vi "Factory1_Main.vi"() -> ()   [LabVIEW 2020]
uses:
  VdDigitalControl_DAQmx_class/VdDigitalControl_DAQmx.lvclass
  VdDigitalControl_AdvantechADAM_class/VdDigitalControl_AdvantechADAM.lvclass
  VdDigitalControl_Simulated_class/VdDigitalControl_Simulated.lvclass
  VdAnalogInput_Simulated_class/VdAnalogInput_Simulated.lvclass
  VdAnalogInput_DAQmx_class/VdAnalogInput_DAQmx.lvclass
  VdDigitalControl_class/VdDigitalControl.lvclass
  VdAnalogInput_class/VdAnalogInput.lvclass
  VdInstrument_class/VdInstrument.lvclass
panel:
  out "Voltages":cluster{"[0]":dbl, "[1]":dbl}(graph)
  out "error out":errorcluster
  out "CurrentState":bool[](array[boolean])
  # "<< Pump\n<< Fan"
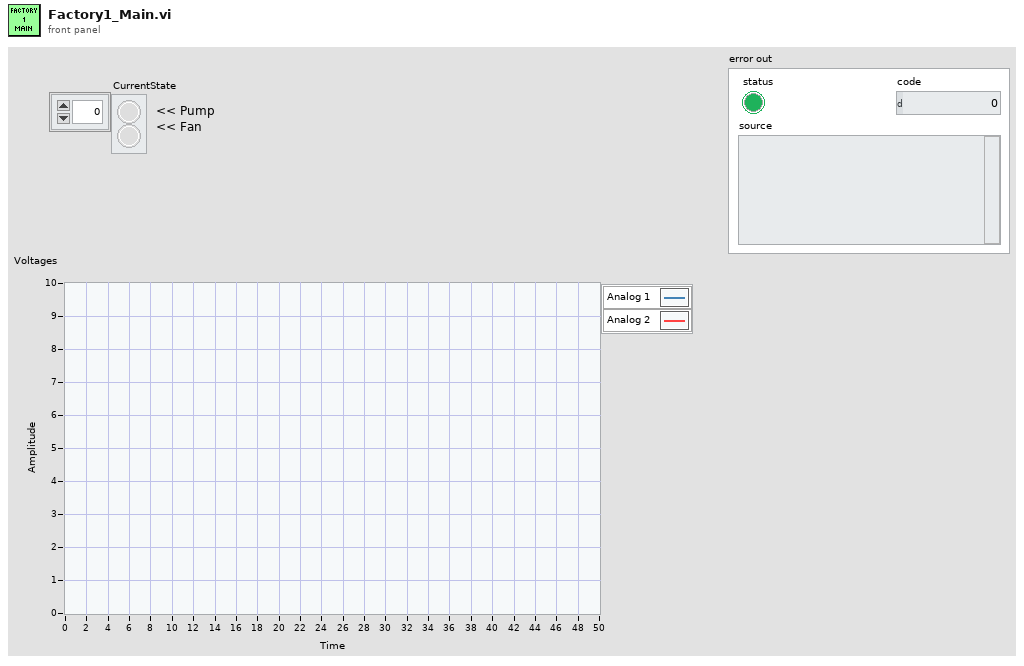
[diagram p1: front panel]
types:
  T1 = cluster{"VdDigitalControl_DAQmx":refnum<class "VdDigitalControl_DAQmx.lvclass">, "VdDigitalControl_AdvantechADAM":refnum<class "VdDigitalControl_AdvantechADAM.lvclass">, "VdDigitalControl_Simulated":refnum<class "VdDigitalControl_Simulated.lvclass">, "VdAnalogInput_Simulated":refnum<class "VdAnalogInput_Simulated.lvclass">, "VdAnalogInput_DAQmx":refnum<class "VdAnalogInput_DAQmx.lvclass">}
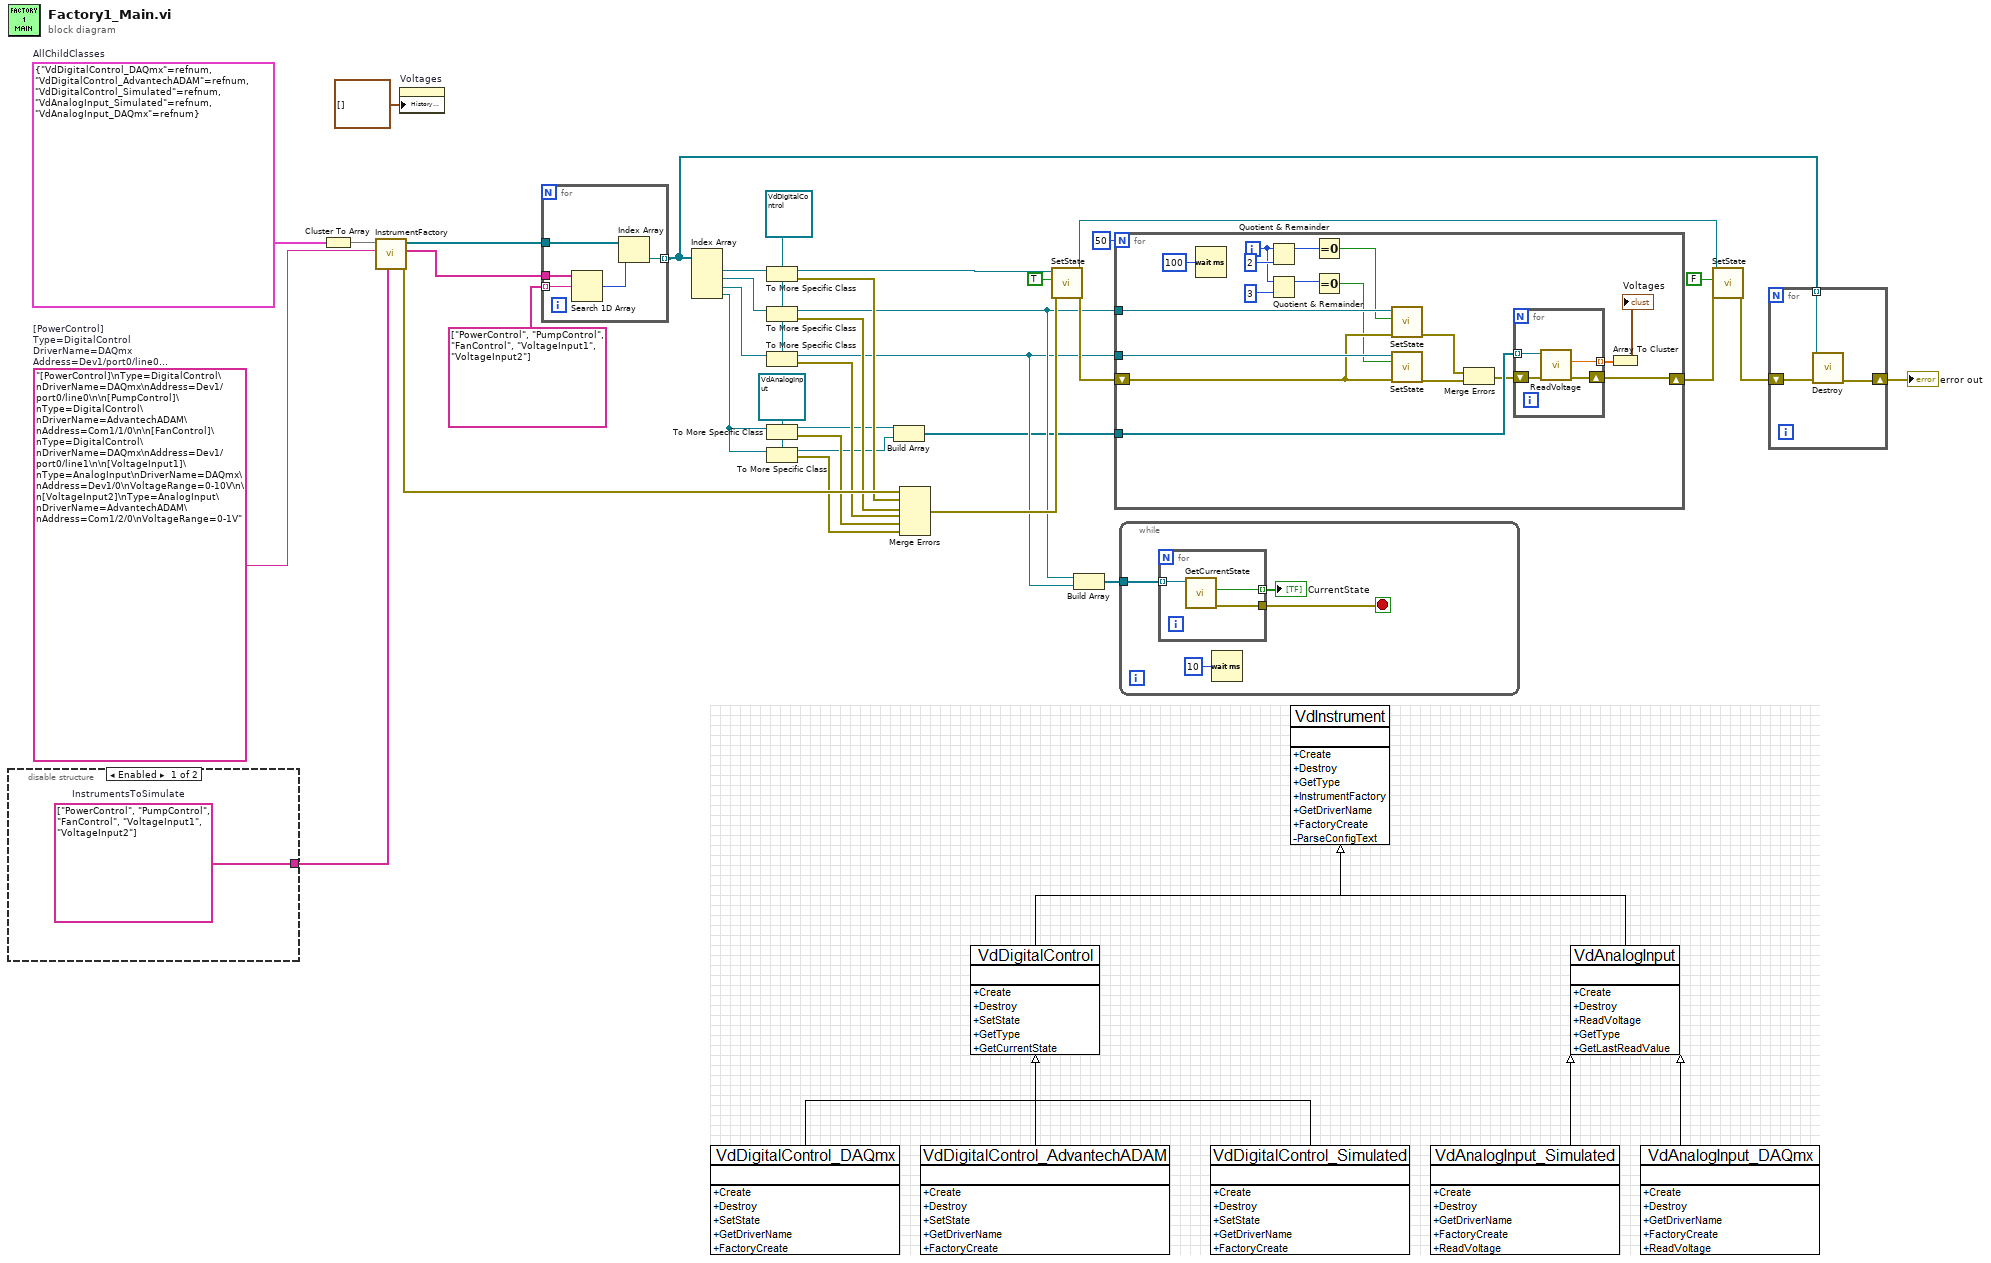
[diagram p0: block diagram]
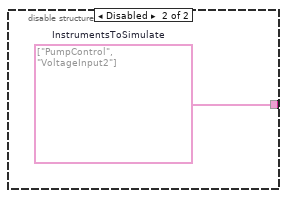
[diagram p2: hidden frame]
diagram:
  w11 = refnum<class "VdAnalogInput.lvclass"> refnum ("VdAnalogInput")
  w25 = refnum<class "VdDigitalControl.lvclass"> refnum ("VdDigitalControl")
  w35 = "[PowerControl]\nType=DigitalControl\nDriverName=DAQmx\nAddress=Dev1/port0/line0\n\n[PumpControl]\nType=DigitalControl\nDriverName=AdvantechADAM\nAddress=Com1/1/0\n\n[FanControl]\nType=DigitalControl\nDriverName=DAQmx\nAddress=Dev1/port0/line1\n\n[VoltageInput1]\nType=AnalogInput\nDriverName=DAQmx\nAddress=Dev1/0\nVoltageRange=0-10V\n\n[VoltageInput2]\nType=AnalogInput\nDriverName=AdvantechADAM\nAddress=Com1/2/0\nVoltageRange=0-1V"  # [PowerControl] Type=DigitalControl DriverName=DAQmx Address=Dev1/port0/line0  [PumpControl] Type=DigitalControl DriverName=AdvantechADAM Address=Com1/1/0  [FanControl] Type=DigitalControl DriverName=DAQmx Address=Dev1/port0/line1  [VoltageInput1] Type=AnalogInput DriverName=DAQmx Address=Dev1/0 VoltageRange=0-10V  [VoltageInput2] Type=AnalogInput DriverName=AdvantechADAM Address=Com1/2/0 VoltageRange=0-1V
  w36 = T1 {"VdDigitalControl_DAQmx"=refnum, "VdDigitalControl_AdvantechADAM"=refnum, "VdDigitalControl_Simulated"=refnum, "VdAnalogInput_Simulated"=refnum, "VdAnalogInput_DAQmx"=refnum}  # AllChildClasses
  n1 = disable-structure shown="Enabled" {
    disable-tunnel: [w38 w39] -> w34
    frame Enabled {
      w38 = string[] ["PowerControl", "PumpControl", "FanControl", "VoltageInput1", "VoltageInput2"]  # InstrumentsToSimulate
    }
    frame Disabled {
      w39 = string[] ["PumpControl", "VoltageInput2"]  # InstrumentsToSimulate
    }
  }
  n2 = Cluster To Array(cluster=w36) -> (array=w37:refnum<class "VdInstrument.lvclass">[])
  n3 = call "InstrumentFactory.vi"("InstrumentsToSimulate"=w34, "InstrumentConfig(ini)"=w35, "AllInstrumentDriver"=w37) -> ("error out"=w23:errorcluster, "InstrumentNamesCreated"=w32:string[], "InstrumentCreated"=w33:refnum<class "VdInstrument.lvclass">[])  [unwired: 6 in]
  n4 = property on="Voltages" class="WFChart (strict)"("History Data"=cluster{"[0]":dbl, "[1]":dbl}[] []) -> ()  [unwired: 2 in, 2 out]
  n5 = for {
    tunnel: w33 -> [w44]
    tunnel: w32 -> [w43]
    tunnel: string[] ["PowerControl", "PumpControl", "FanControl", "VoltageInput1", "VoltageInput2"] -> [w41] mode=indexing
    tunnel: [w40] -> w14 mode=indexing
    n6 = Search 1D Array(1D array=w43, element=w41) -> (index of element=w42:i32)  [unwired: 1 in]
    n7 = Index Array(array=w44, index=w42) -> (element=w40:refnum<class "VdInstrument.lvclass">)
  }
  n8 = Index Array(array=w14) -> (element #1=w30:refnum<class "VdInstrument.lvclass">, element #2=w29:refnum<class "VdInstrument.lvclass">, element #3=w26:refnum<class "VdInstrument.lvclass">, element #4=w12:refnum<class "VdInstrument.lvclass">)  [unwired: 4 in]
  n9 = To More Specific Class(target class=w25, reference=w30) -> (specific class reference=w28:refnum<class "VdDigitalControl.lvclass">, error out=w21:errorcluster)  [unwired: 1 in]
  n10 = To More Specific Class(target class=w25, reference=w29) -> (specific class reference=w17:refnum<class "VdDigitalControl.lvclass">, error out=w20:errorcluster)  [unwired: 1 in]
  n11 = To More Specific Class(target class=w25, reference=w26) -> (specific class reference=w16:refnum<class "VdDigitalControl.lvclass">, error out=w19:errorcluster)  [unwired: 1 in]
  n12 = To More Specific Class(target class=w11, reference=w12) -> (specific class reference=w8:refnum<class "VdAnalogInput.lvclass">, error out=w10:errorcluster)  [unwired: 1 in]
  n13 = To More Specific Class(target class=w11, reference=w12) -> (specific class reference=w7:refnum<class "VdAnalogInput.lvclass">, error out=w9:errorcluster)  [unwired: 1 in]
  n14 = Build Array(w8, w7) -> (w6:refnum<class "VdAnalogInput.lvclass">[])
  n15 = Merge Errors(w23, w21, w20, w19, w10, w9) -> (w22:errorcluster)
  n16 = call-dynamic "SetState.vi"("Error In"=w22, "State"=TRUE, "reference in"=w28) -> ("Error Out"=w24:errorcluster, "reference in"=w1:refnum<class "VdDigitalControl.lvclass">)  [unwired: 7 in]
  n17 = Build Array(w17, w16) -> (w15:refnum<class "VdDigitalControl.lvclass">[])
  n18 = for {
    N: 50 -> [_]
    tunnel: w17 -> [w62]
    tunnel: w16 -> [w61]
    shift-right: [w49] -> w4
    shift-left: w24 -> [w60]
    tunnel: w6 -> [w53]
    i -> [w48]
    n19 = Wait (ms)(milliseconds to wait=u32 100) -> ()  [unwired: 1 out]
    n20 = Quotient & Remainder(x=w48, y=2) -> (x-y*floor(x/y)=w55:i32)  [unwired: 1 out]
    n21 = Quotient & Remainder(x=w48, y=3) -> (x-y*floor(x/y)=w46:i32)  [unwired: 1 out]
    n22 = Equal To 0?(x=w55) -> (x = 0?=w54:bool)
    n23 = Equal To 0?(x=w46) -> (x = 0?=w45:bool)
    n24 = call-dynamic "SetState.vi"("Error In"=w60, "State"=w54, "reference in"=w62) -> ("Error Out"=w57:errorcluster)  [unwired: 7 in, 1 out]
    n25 = call-dynamic "SetState.vi"("Error In"=w60, "State"=w45, "reference in"=w61) -> ("Error Out"=w58:errorcluster)  [unwired: 7 in, 1 out]
    n26 = Merge Errors(w57, w58) -> (w52:errorcluster)
    n27 = for {
      tunnel: w53 -> [w66] mode=indexing
      shift-right: [w64] -> w49
      shift-left: w52 -> [w65]
      tunnel: [w63] -> w51 mode=indexing
      n28 = call-dynamic "ReadVoltage.vi"("Error In"=w65, "reference in"=w66) -> ("Error Out"=w64:errorcluster, "Voltage"=w63:dbl)  [unwired: 7 in, 1 out]
    }
    n29 = Array To Cluster(array=w51) -> (cluster=→"Voltages":cluster{"[0]":dbl, "[1]":dbl})
  }
  n30 = while {
    tunnel: w15 -> [w70]
    stop <- w68 stop-if-true
    n31 = for {
      tunnel: w70 -> [w73] mode=indexing
      tunnel: [w72] -> w69 mode=indexing
      tunnel: [w71] -> w68
      n32 = call-dynamic "GetCurrentState.vi"("reference in"=w73) -> ("Error Out"=w71:errorcluster, "CurrentState"=w72:bool)  [unwired: 8 in, 1 out]
    }
    "CurrentState" <- w69
    n33 = Wait (ms)(milliseconds to wait=u32 10) -> ()  [unwired: 1 out]
  }
  n34 = call-dynamic "SetState.vi"("Error In"=w4, "State"=FALSE, "reference in"=w1) -> ("Error Out"=w3:errorcluster)  [unwired: 7 in, 1 out]
  n35 = for {
    tunnel: w14 -> [w75] mode=indexing
    shift-right: [w74] -> w13
    shift-left: w3 -> [w76]
    n36 = call-dynamic "Destroy.vi"("Error In"=w76, "reference in"=w75) -> ("Error Out"=w74:errorcluster)  [unwired: 8 in, 1 out]
  }
  "error out" <- w13
